vi "LSX Wait For Axis Stop.vi"(7 "pbATimeout":i32, 8 "error in (no error)":errorcluster, 9 "lATimeoutValue":i32, 10 "lAFlags":i32, 11 "lLSID":i32) -> (0 "error out":errorcluster, 3 "function return":i32, 5 "pbATimeout out":i32)   [LabVIEW 2018, in "Tango.lvlib"]
doc: "TANGOAPI int TANGOCALL LSX_WaitForAxisStop (int lLSID, int lAFlags, int lATimeoutValue, BOOL *pbATimeout);"
uses:
  Tango.lvlib
  SubVIs/Tango_DLL.dll
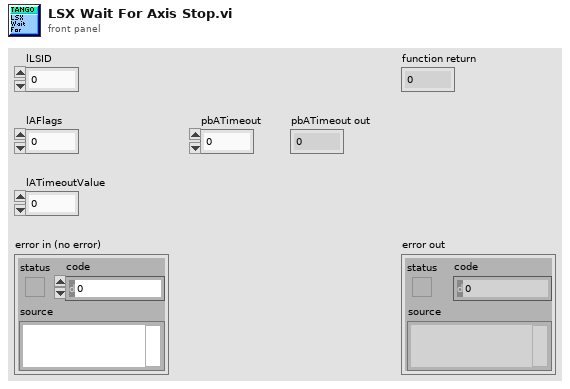
[diagram p1: front panel]
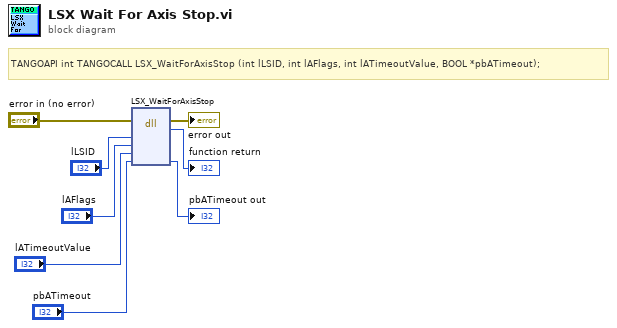
[diagram p0: block diagram]
diagram:
  # "TANGOAPI int TANGOCALL LSX_WaitForAxisStop (int lLSID, int lAFlags, int lATimeoutValue, BOOL *pbATimeout);"
  n1 = dll-call lib="C:/Users/Familie/Documents/LabviewIX81/lib/TANGO Stage/SubVIs/Tango_DLL.*" fn="LSX_WaitForAxisStop"(error in="error in (no error)", "lLSID"="lLSID", "lAFlags"="lAFlags", "lATimeoutValue"="lATimeoutValue", "pbATimeout"="pbATimeout") -> (error out=→"error out":errorcluster, →"function return":i32, "pbATimeout"=→"pbATimeout out":i32)  [unwired: 5 in, 1 out]
